vi "LWXPS_GetPistonState.vi"(1 "XPS Reference IN":refnum<k24>, 4 "LabVIEW error IN":errorcluster) -> (12 "XPS Reference OUT":refnum<k24>, 13 "LabVIEW error OUT":errorcluster, 14 "Returned error code":i32, 15 "Command State":i32, 16 "Piston limit Down":i32, 17 "Piston limit Up":i32, 18 "Lift Pin UP Interlock":i32, 19 "XPS Error String":string)   [LabVIEW 2014]
uses:
  D:/XPSQ8_LabView_Library/Development/Source/Dll/Newport.XPS.CommandInterface.dll
  Dll/Newport.XPS.CommandInterface.dll
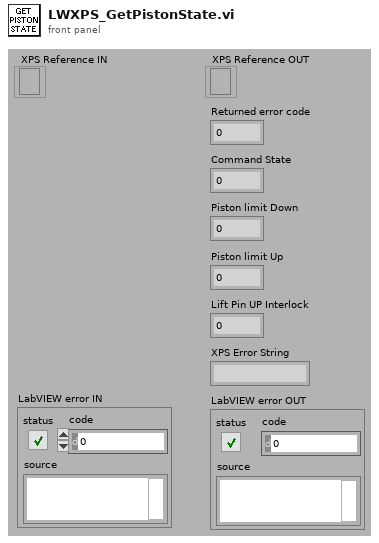
[diagram p1: front panel]
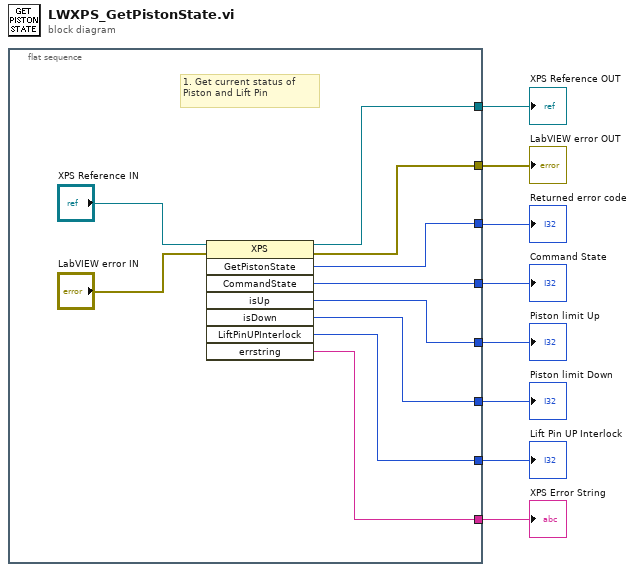
[diagram p0: block diagram]
diagram:
  n1 = flat-sequence {
    tunnel: [w17] -> w8
    tunnel: [w16] -> w7
    tunnel: [w15] -> w6
    tunnel: [w13] -> w4
    tunnel: [w12] -> w3
    tunnel: [w11] -> w2
    tunnel: [w10] -> w1
    tunnel: [w9] -> w5
    frame #0 {
      # "1. Get current status of Piston and Lift Pin"
      n2 = invoke class="XPS" method="GetPistonState"(reference="XPS Reference IN", error in="LabVIEW error IN") -> (reference out=w17:refnum<k24>, error out=w16:errorcluster, "GetPistonState"=w15:i32, "CommandState"=w13:i32, "isUp"=w12:i32, "isDown"=w11:i32, "LiftPinUPInterlock"=w10:i32, "errstring"=w9:string)  [unwired: 6 in]
    }
  }
  "XPS Reference OUT" <- w8
  "LabVIEW error OUT" <- w7
  "Returned error code" <- w6
  "XPS Error String" <- w5
  "Command State" <- w4
  "Piston limit Up" <- w3
  "Piston limit Down" <- w2
  "Lift Pin UP Interlock" <- w1
